vi "SVPO Limit Testing (1 Ch) (SGL Array).vi"(7 "reset? (F)":bool, 9 "lower limit":sgl=-inf format="%.2f", 10 "upper limit":sgl=inf format="%.2f", 11 "signal in":sgl[](array[numeric])) -> (1 "lower limit clearance":sgl format="%.6f", 2 "upper limit clearance":sgl format="%.6f", 3 "test passed?":bool)   [LabVIEW 2017, in "SoundVib_LimitTest.lvlib"]
doc: "Performs limit testing on single-precision waveforms, single-precision scaled arrays, or double-precision scalar measurements. You can specify an upper and lower boundary of the envelope to define a pass range. This VI uses the defined pass range to test the input signal. VI outputs apply to all the tests since the last VI reset. Use this VI on embedded targets that have limited computational resources. Wire data to the <B>value in</B> input to determine the polymorphic instance to use or manually select the instance."
uses:
  <vilib>/addons/Sound and Vibration/svt_Limit Test/SoundVib_LimitTest.lvlib
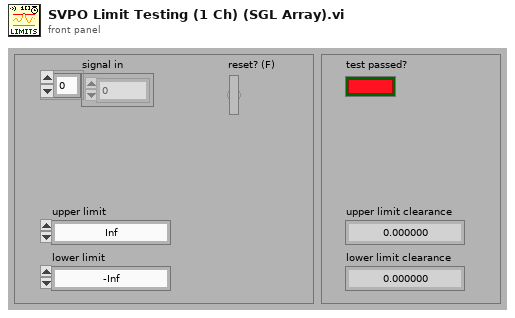
[diagram p1: front panel]
types:
  T1 = typedef "svc_SGL Limit State.ctl" = cluster{"upper limit clearance":sgl, "lower limit clearance":sgl, "test passed?":bool, "block passed?":bool}
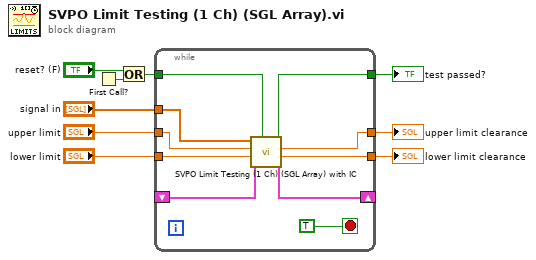
[diagram p0: block diagram]
diagram:
  n1 = First Call?() -> (First Call?: T/F=w6:bool)
  n2 = Or(x="reset? (F)", y=w6) -> (x .or. y?=w7:bool)
  n3 = while {
    tunnel: "upper limit" -> [w17]
    tunnel: "lower limit" -> [w16]
    tunnel: w7 -> [w11]
    tunnel: "signal in" -> [w18]
    shift-right: [w15] -> _
    shift-left: _ -> [w14]
    tunnel: [w13] -> w3
    tunnel: [w12] -> w2
    tunnel: [w10] -> w1
    stop <- TRUE stop-if-true
    n4 = call <vilib>:"SVPO Limit Testing (1 Ch) (SGL Array) with IC.vi"("reset? (F)"=w11, "initial conditions"=w14, "lower limit"=w16, "upper limit"=w17, "signal in"=w18) -> ("final conditions"=w15:T1, "lower limit clearance"=w13:sgl, "upper limit clearance"=w12:sgl, "test passed?"=w10:bool)  [unwired: 3 in]
  }
  "test passed?" <- w1
  "upper limit clearance" <- w2
  "lower limit clearance" <- w3
